vi "fftw__plan_dft_r2c_1d_poly.vi"   [LabVIEW 2020, in "FFTWDLL.lvlib"]
doc: "Make a FFTW plan for 1D real-to-cplx forward transform."
uses:
  FFTWDLL.lvlib
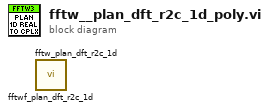
[diagram p0: block diagram]
diagram:
  n1 = call "fftwf_plan_dft_r2c_1d.vi"() -> ()  [unwired: 8 in, 4 out]
  n2 = call "fftw_plan_dft_r2c_1d.vi"() -> ()  [unwired: 8 in, 4 out]
